vi "XYZTWaveforms.vi"(3 "Microscope Settings":T2={"Mode"=enum."XYZT", "Slit"={"Scanning Mode"=0.0, "Slit Width /%"=0.0}, "Colour"=[], "Exposure/ms"=40.0, "Piezo Position /um"=10.0, "ROI"={"X"={"Start /px"=0.0, "Step /px"=0.0, "Range /px"=2048.0}, "Y"={"Start /px"=0.0, "Step /px"=0.0, "Range /px"=0.0}, "Z "={"Start /um"=0.0, "Step/um"=10.0, "Range /um"=100.0}, "T "={"Start /s"=0.0, "Step /s"=1.0, "Range /s"=60.0}}, "Samples per millisecond"=100.0, "Relax/ms"=10.0, "Readout Direction"=0.0, "Trigger Source"=0.0, "Camera Delay /ms"=11.0, "Under Scan /ms"=5.0, "Calibration Coordinates"={"Top Left"=[], "Top Right"=[], "Bottom Left"=[], "Bottom Right"=[], "Waveforms"={"Analogue Out"=[], "Digital Out"=[]}}} {"Under Scan /ms" min=0.0 max=10.0 step=0.05; "ROI"."T"."Range /s" min=0.0 max=10.0 step=0.05; "ROI"."T"."Step /s" min=0.0 max=10.0 step=0.05; "ROI"."T"."Start /s" min=0.0 max=10.0 step=0.05; "ROI"."X"."Range /px" min=0.0 max=10.0 step=0.05; "ROI"."X"."Step /px" min=0.0 max=10.0 step=0.05; "ROI"."X"."Start /px" min=0.0 max=10.0 step=0.05; "ROI"."Y"."Range /px" min=0.0 max=10.0 step=0.05; "ROI"."Y"."Step /px" min=0.0 max=10.0 step=0.05; "ROI"."Y"."Start /px" min=0.0 max=10.0 step=0.05; "ROI"."Z"."Range /um" min=0.0 max=10.0 step=0.05; "ROI"."Z"."Step/um" min=0.0 max=10.0 step=0.05; "ROI"."Z"."Start /um" min=0.0 max=10.0 step=0.05; "Colour"."Filter" items=["Empty"=1, ""=2, ""=3, "561"=4, ""=5, "488"=6]; "Camera Delay /ms" min=0.0 max=10.0 step=0.05; "Trigger Source" items=["Internal"=1.0, "External"=2.0]; "Readout Direction" items=["Forward"=1.0, "Backward"=2.0]; "Slit"."Scanning Mode" items=["Full Frame"=1.0, "Slit Scanning"=12.0]; "Piezo Position /um" min=0.0 max=10.0 step=0.05}) -> (0 "Digital Out":digitalwaveform[](array[waveform]), 1 "Analogue Out":waveform(dbl)[](array[waveform]))   [LabVIEW 2016]
uses:
  <vilib>/Waveform/WDTOps.llb/WDT Append Waveforms DBL.vi
  <vilib>/Waveform/DWDTOps.llb/DWDT Append Digital Samples.vi
  <vilib>/Waveform/WDTOps.llb/WDT Waveform Duration DBL.vi
  controls/Microscope Settings.ctl
panel:
  out "Mixed Signal Graph 3":T1(graph)
  out "duration":dbl format="%0.2f"
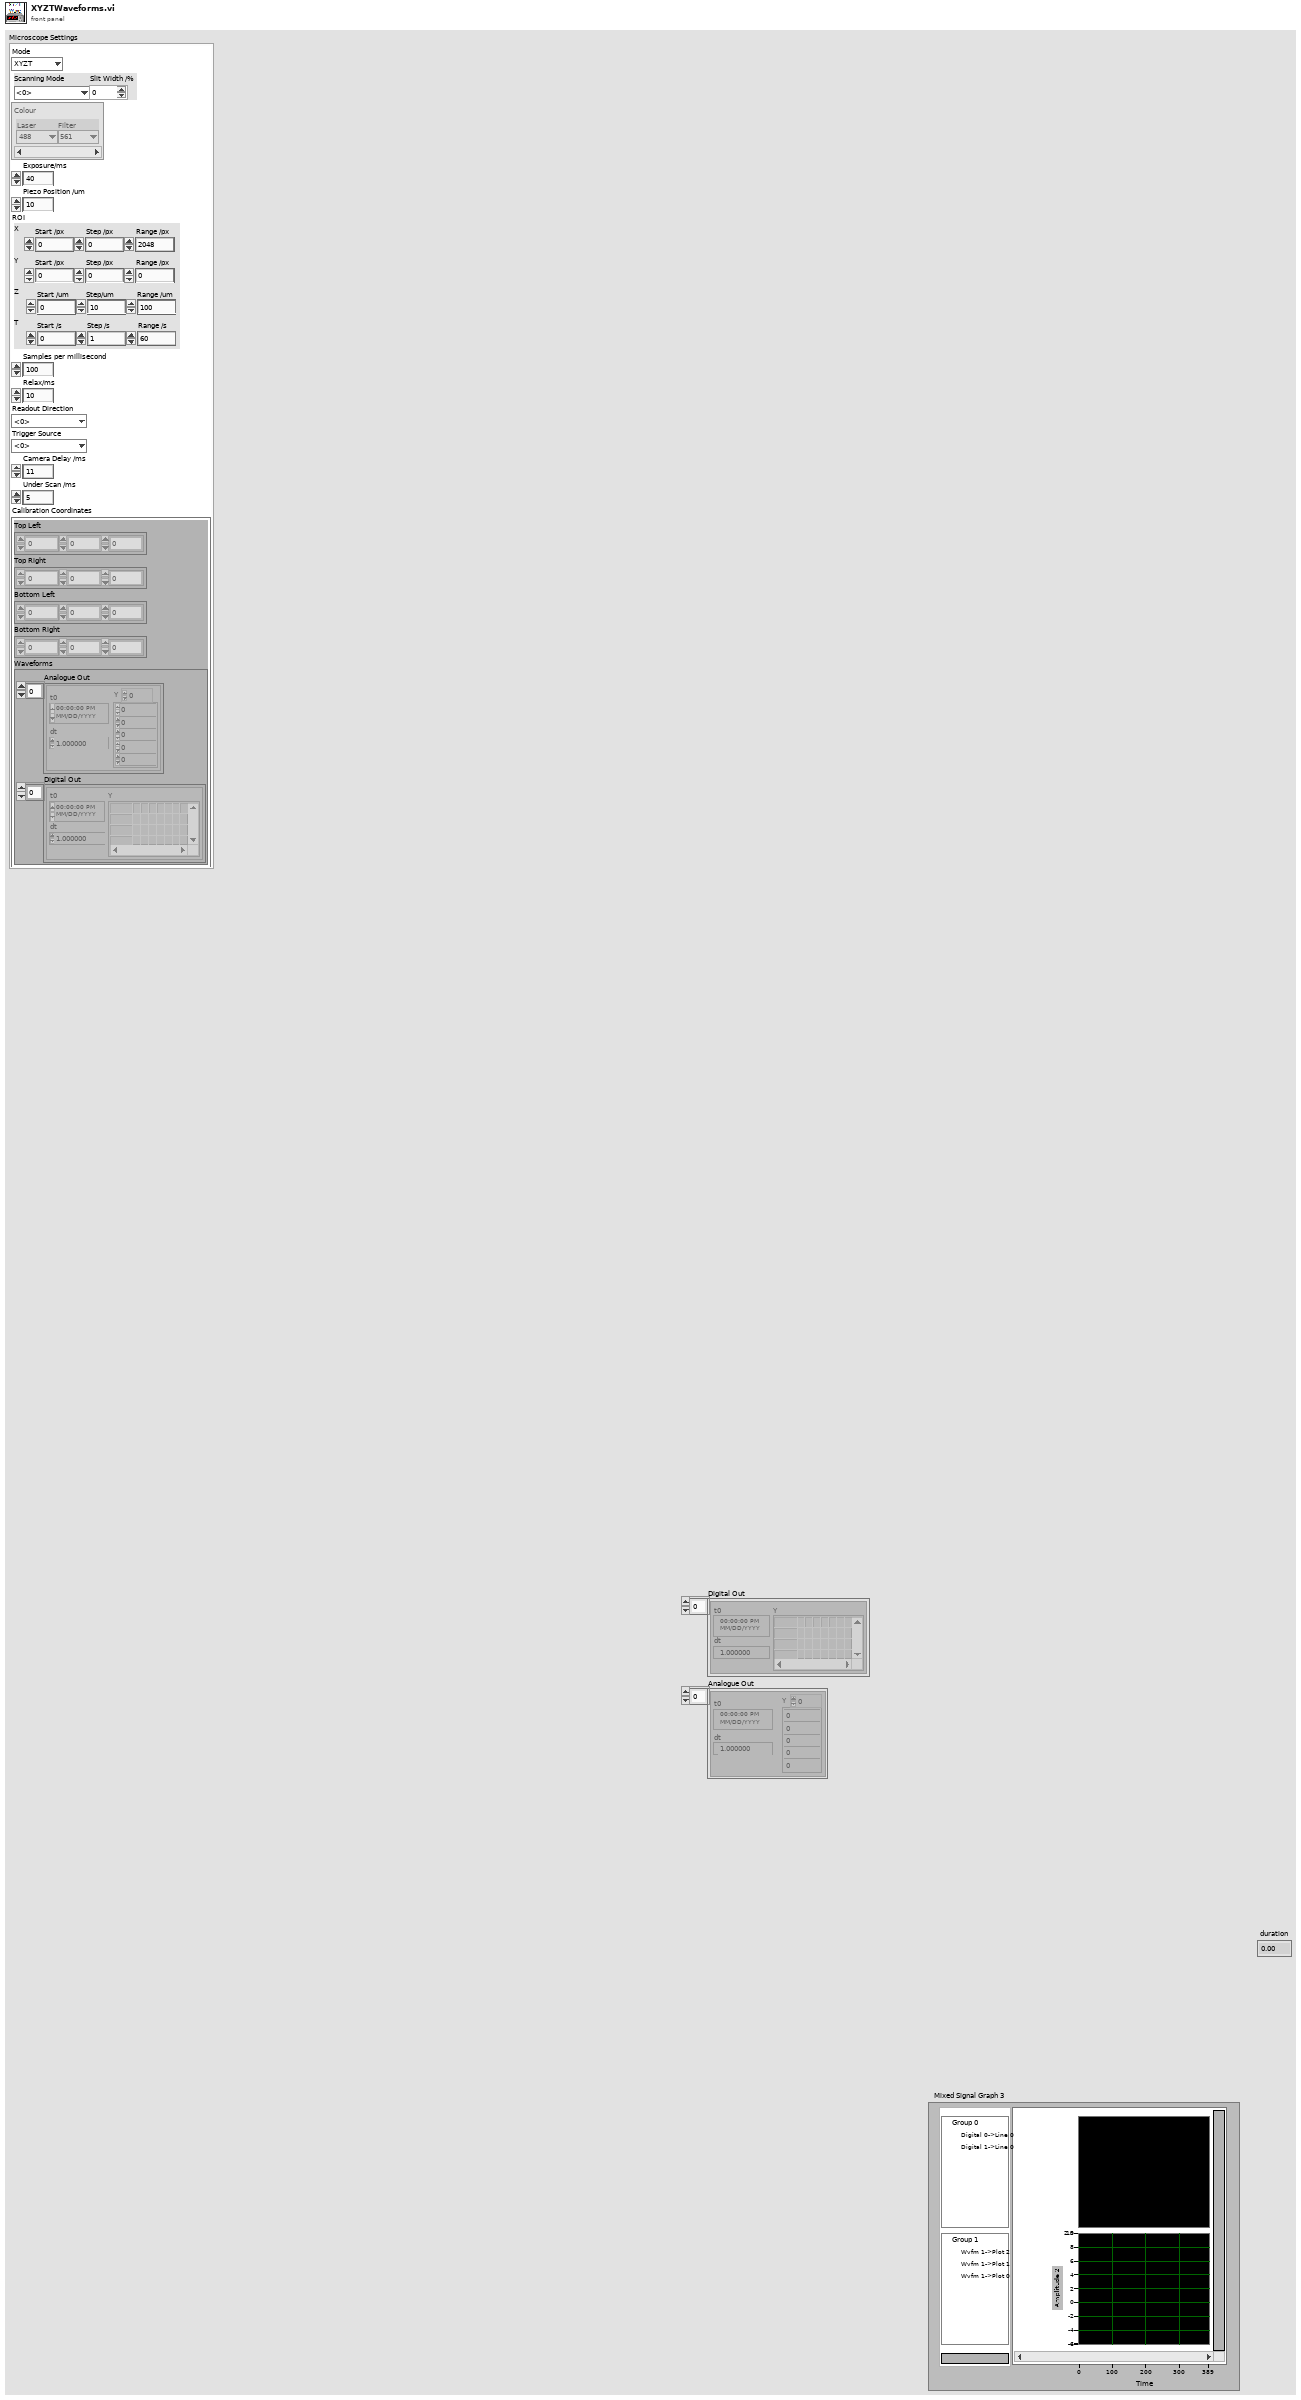
[diagram p1: front panel]
types:
  T1 = cluster{"Digital Out out":digitalwaveform[], "Analogue Out out":waveform(dbl)[]}
  T2 = typedef "Microscope Settings.ctl" = cluster{"Mode":enum16{"Brightfield", "X", "XY", "XYZ", "XYZT", "XYZC", "Tweezers", "Virus"}, "Slit":cluster{"Scanning Mode":dbl, "Slit Width /%":dbl}, "Colour":cluster{"Laser":enum16{"Brightfield", "445", "488", "561", "647"}, "Filter":u16}[], "Exposure/ms":dbl, "Piezo Position /um":dbl, "ROI":cluster{"X":cluster{"Start /px":dbl, "Step /px":dbl, "Range /px":dbl}, "Y":cluster{"Start /px":dbl, "Step /px":dbl, "Range /px":dbl}, "Z ":cluster{"Start /um":dbl, "Step/um":dbl, "Range /um":dbl}, "T ":cluster{"Start /s":dbl, "Step /s":dbl, "Range /s":dbl}}, "Samples per millisecond":dbl, "Relax/ms":dbl, "Readout Direction":dbl, "Trigger Source":dbl, "Camera Delay /ms":dbl, "Under Scan /ms":dbl, "Calibration Coordinates":cluster{"Top Left":dbl[], "Top Right":dbl[], "Bottom Left":dbl[], "Bottom Right":dbl[], "Waveforms":cluster{"Analogue Out":waveform(dbl)[], "Digital Out":digitalwaveform[]}}}
  T3 = cluster{"Start /s":dbl, "Step /s":dbl, "Range /s":dbl}
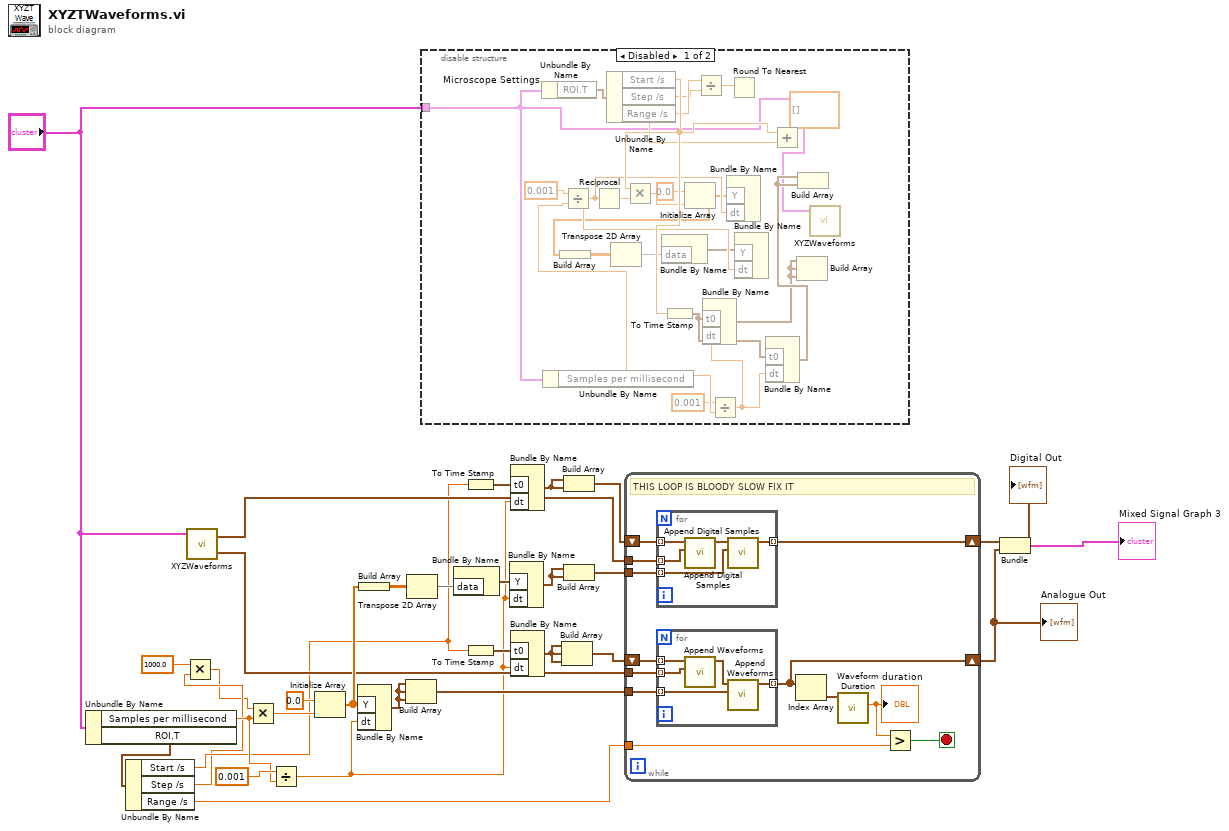
[diagram p0: block diagram]
diagram:
  n1 = Unbundle By Name("Microscope Settings") -> ("Samples per millisecond"=w9:dbl, "ROI.T"=w7:T3)
  n2 = Unbundle By Name(w7) -> ("Start /s"=w5:dbl, "Step /s"=w3:dbl, "Range /s"=w4:dbl)
  n3 = Multiply(x=1000.0, y=w3) -> (x*y=w2:dbl)
  n4 = call "XYZWaveforms.vi"("Microscope Settings"="Microscope Settings") -> ("Analogue Out out"=w14:waveform(dbl)[], "Digital Out out"=w15:digitalwaveform[])  [unwired: 2 in]
  n5 = Multiply(x=w2, y=w9) -> (x*y=w23:dbl)
  n6 = Divide(x=0.001 ("element"), y=w9) -> (x/y=w8:dbl)
  n7 = Initialize Array(0.0 ("element"), w23) -> (w22:dbl[])
  n8 = Bundle By Name("Y"=w22, "dt"=w8) -> (w25:waveform(dbl))  [unwired: 1 in]
  n9 = Build Array(w22) -> (w21:dbl[][])
  n10 = Build Array(w25, w25, w25) -> (w16:waveform(dbl)[])
  n11 = Transpose 2D Array(2D array=w21) -> (transposed array=w20:dbl[][])
  n12 = disable-structure shown="Disabled" {
    disable-tunnel: "Microscope Settings" -> [w32 _]
    frame Disabled {
      (unwired) dbl[][] []
      n13 = Unbundle By Name(w32) -> ("ROI.T"=w35:T3)
      n14 = Unbundle By Name(w32) -> ("Samples per millisecond"=w52:dbl)
      n15 = Divide(x=0.001 ("y"), y=w52) -> (x/y=w44:dbl)
      n16 = Reciprocal(x=w44) -> (1/x=w37:dbl)
      n17 = Unbundle By Name(w35) -> ("Start /s"=w47:dbl, "Step /s"=w45:dbl, "Range /s"=w46:dbl)
      n18 = Multiply(x=w47, y=w37) -> (x*y=w39:dbl)
      n19 = To Time Stamp(1:w47) -> (0:w49:timestamp)
      n20 = Initialize Array(0.0 ("element"), w39) -> (w42:dbl[])
      n21 = Build Array(w42) -> (w40:dbl[][])
      n22 = Transpose 2D Array(2D array=w40) -> (transposed array=w41:dbl[][])
      n23 = Bundle By Name("data"=w41) -> (w43:digitaldata)  [unwired: 1 in]
      n24 = Divide(x=w46, y=w45) -> (x/y=w34:dbl)
      n25 = Divide(x=0.001 ("y"), y=w52) -> (x/y=w33:dbl)
      n26 = Bundle By Name("t0"=w49, "dt"=w33) -> (w48:waveform(dbl))  [unwired: 1 in]
      n27 = Bundle By Name("Y"=w42, "dt"=w44) -> ()  [unwired: 1 in, 1 out]
      n28 = Round To Nearest(number=w34) -> ()  [unwired: 1 out]
      n29 = Bundle By Name("Y"=w43, "dt"=w44) -> ()  [unwired: 1 in, 1 out]
      n30 = Bundle By Name("t0"=w49, "dt"=w33) -> (w50:digitalwaveform)  [unwired: 1 in]
      n31 = Add(x=w47, y=w46) -> ()  [unwired: 1 out]
      n32 = Build Array(w48, w48, w48) -> ()  [unwired: 1 out]
      n33 = Build Array(w50, w50) -> ()  [unwired: 1 out]
      n34 = call "XYZWaveforms.vi"("Microscope Settings"=w32) -> ()  [unwired: 2 in, 2 out]
    }
    frame Enabled {
    }
  }
  n35 = Bundle By Name("data"=w20) -> (w19:digitaldata)  [unwired: 1 in]
  n36 = To Time Stamp(1:w5) -> (0:w31:timestamp)
  n37 = To Time Stamp(1:w5) -> (0:w26:timestamp)
  n38 = Bundle By Name("Y"=w19, "dt"=w8) -> (w18:digitalwaveform)  [unwired: 1 in]
  n39 = Bundle By Name("t0"=w31, "dt"=w8) -> (w30:digitalwaveform)  [unwired: 1 in]
  n40 = Bundle By Name("t0"=w26, "dt"=w8) -> (w27:waveform(dbl))  [unwired: 1 in]
  n41 = Build Array(w27, w27, w27) -> (w28:waveform(dbl)[])
  n42 = Build Array(w30, w30) -> (w29:digitalwaveform[])
  n43 = Build Array(w18, w18) -> (w17:digitalwaveform[])
  n44 = while {
    shift-right: [w59] -> w11
    shift-left: w28 -> [w64]
    shift-right: [w62] -> w12
    shift-left: w29 -> [w63]
    tunnel: w17 -> [w61]
    tunnel: w16 -> [w60]
    tunnel: w4 -> [w56]
    tunnel: w15 -> [w55]
    tunnel: w14 -> [w54]
    stop <- w53 stop-if-true
    # "THIS LOOP IS BLOODY SLOW FIX IT"
    n45 = for {
      tunnel: w55 -> [w68] mode=indexing
      tunnel: w63 -> [w69] mode=indexing
      tunnel: [w65] -> w62 mode=indexing
      tunnel: w61 -> [w66] mode=indexing
      n46 = call-poly <vilib>:"Append Digital Samples.vi"("digital waveform B"=w68, "digital waveform A"=w69) -> ("digital waveform out"=w67:digitalwaveform)  [unwired: 8 in, 1 out]
      n47 = call-poly <vilib>:"Append Digital Samples.vi"("digital waveform B"=w66, "digital waveform A"=w67) -> ("digital waveform out"=w65:digitalwaveform)  [unwired: 8 in, 1 out]
    }
    n48 = for {
      tunnel: w54 -> [w73] mode=indexing
      tunnel: w64 -> [w74] mode=indexing
      tunnel: [w71] -> w59 mode=indexing
      tunnel: w60 -> [w70] mode=indexing
      n49 = call-poly <vilib>:"Append Waveforms.vi"("waveform B"=w73, "waveform A"=w74) -> ("waveform out"=w72:waveform(dbl))  [unwired: 8 in, 1 out]
      n50 = call-poly <vilib>:"Append Waveforms.vi"("waveform B"=w70, "waveform A"=w72) -> ("waveform out"=w71:waveform(dbl))  [unwired: 8 in, 1 out]
    }
    n51 = Index Array(array=w59) -> (element=w58:waveform(dbl))  [unwired: 1 in]
    n52 = call-poly <vilib>:"Waveform Duration.vi"("waveform in"=w58) -> ("duration"=w57:dbl)  [unwired: 8 in, 2 out]
    "duration" <- w57
    n53 = Greater?(x=w57, y=w56) -> (0:w53:bool)
  }
  "Digital Out" <- w12
  "Analogue Out" <- w11
  n54 = Bundle(w12, w11) -> (→"Mixed Signal Graph 3":cluster{digitalwaveform[], waveform(dbl)[]})  [unwired: 1 in]
